vi "Check 2D Limits.vi"(2 "error in":T2, 4 "Z-Axis Communications Config":T1={"GPIB address"=22, "GPIB bus"=0, "connection ID"=refnum, "IP"="192.168.2.200", "Active Comm Interface"=0, "Serial Port"="", "Programmer Type"=0} {"Programmer Type" items=["Model 430", "Model 420"]; "Active Comm Interface" items=["TCP/IP (Model 430 Only)", "RS232", "IEEE488"]}, 5 "Y-Axis Communications Config":T1={"GPIB address"=22, "GPIB bus"=0, "connection ID"=refnum, "IP"="192.168.2.200", "Active Comm Interface"=0, "Serial Port"="", "Programmer Type"=0} {"Programmer Type" items=["Model 430", "Model 420"]; "Active Comm Interface" items=["TCP/IP (Model 430 Only)", "RS232", "IEEE488"]}, 6 "Z-Axis Field (T)":dbl format="%.3f", 7 "Y-Axis Field (T)":dbl format="%.3f") -> (0 "Within Limits?":bool, 1 "error out":T2)   [LabVIEW 2016]
uses:
  Instrument_Setup.vi
panel:
  out "Set Magnitude":dbl format="%#_13g"
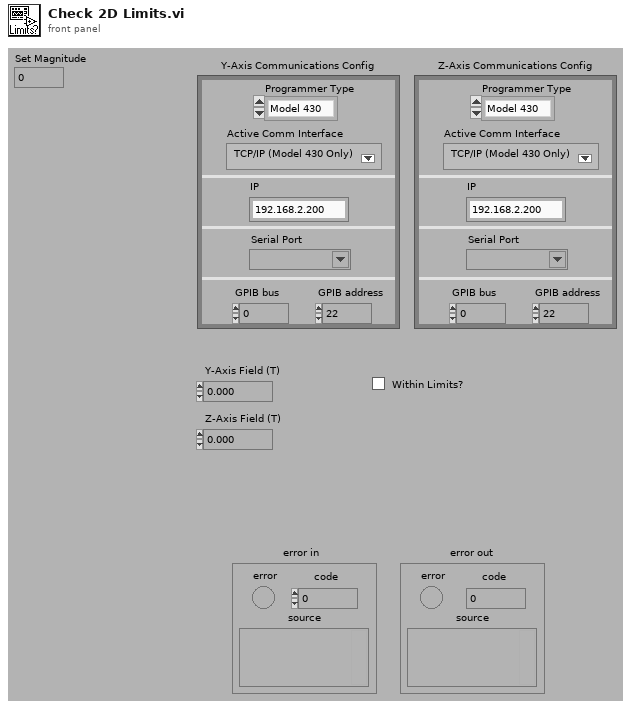
[diagram p1: front panel]
types:
  T1 = cluster{"GPIB address":i16, "GPIB bus":i16, "connection ID":refnum<k5>, "IP":string, "Active Comm Interface":u16, "Serial Port":refnum<visa-resource-name>, "Programmer Type":u16}
  T2 = cluster{"error":bool, "code":i32, "source":string}
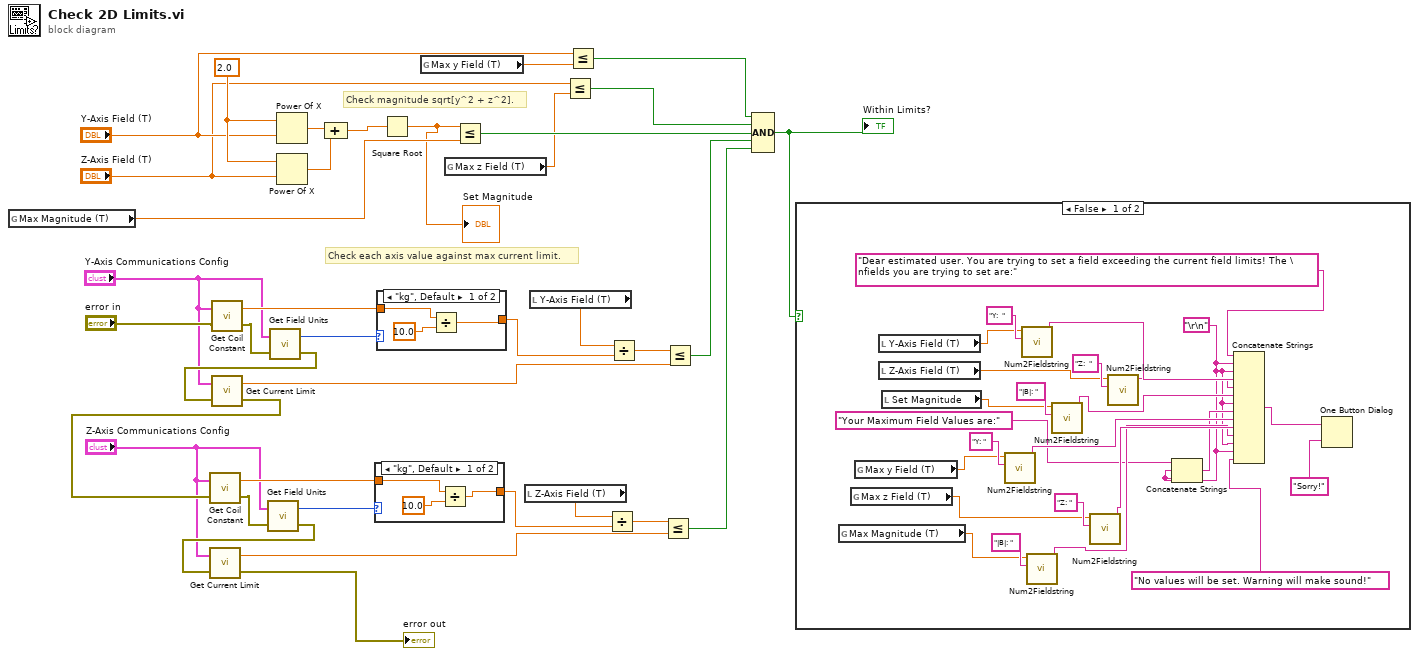
[diagram p0: block diagram]
diagram:
  w37 = 2.0 ("x")
  # "Check each axis value against max current limit."
  # "Check magnitude sqrt[y^2 + z^2]."
  n1 = global read "Instrument_Setup.vi" "Max Magnitude (T)"() -> (w5:dbl)
  n2 = call "Get Coil Constant.vi"("error in"="error in", "Communications Config"="Y-Axis Communications Config") -> ("error out"=w24:T2, "Coil Constant"=w25:dbl)
  n3 = call "Get Field Units.vi"("error in"=w24, "Z-Axis Communications Config"="Y-Axis Communications Config") -> ("error out"=w23:T2, "Field Units"=w26:enum16{"kg", "t"})
  n4 = call "Get Current Limit.vi"("error in"=w23, "Communications Config"="Y-Axis Communications Config") -> ("error out"=w18:T2, "Current Limit (A)"=w16:dbl)
  n5 = call "Get Coil Constant.vi"("error in"=w18, "Communications Config"="Z-Axis Communications Config") -> ("error out"=w20:T2, "Coil Constant"=w21:dbl)
  n6 = call "Get Field Units.vi"("error in"=w20, "Z-Axis Communications Config"="Z-Axis Communications Config") -> ("error out"=w19:T2, "Field Units"=w22:enum16{"kg", "t"})
  n7 = call "Get Current Limit.vi"("error in"=w19, "Communications Config"="Z-Axis Communications Config") -> ("error out"=→"error out":T2, "Current Limit (A)"=w14:dbl)
  n8 = Power Of X(1:"Y-Axis Field (T)", 2:w37) -> (0:w36:dbl)
  n9 = Power Of X(1:"Z-Axis Field (T)", 2:w37) -> (0:w35:dbl)
  n10 = Compound Arithmetic op=ADD(w36, w35) -> (w27:dbl)
  n11 = case shown="\"kg\", Default" w22 {
    tunnel: w21 -> [w39 w41]
    tunnel: [w38 w41] -> w15
    frame "kg", Default {
      n12 = Divide(x=w39, y=10.0) -> (x/y=w38:dbl)
    }
    frame "t" {
    }
  }
  n13 = case shown="\"kg\", Default" w26 {
    tunnel: w25 -> [w44 w45]
    tunnel: [w43 w45] -> w17
    frame "kg", Default {
      n14 = Divide(x=w44, y=10.0) -> (x/y=w43:dbl)
    }
    frame "t" {
    }
  }
  n15 = Square Root(x=w27) -> (sqrt(x)=w1:dbl)
  "Set Magnitude" <- w1
  n16 = global read "Instrument_Setup.vi" "Max y Field (T)"() -> (w3:dbl)
  n17 = global read "Instrument_Setup.vi" "Max z Field (T)"() -> (w4:dbl)
  n18 = Less Or Equal?(x=w1, y=w5) -> (x <= y?=w30:bool)
  n19 = local read "Z-Axis Field (T)"() -> (w31:dbl)
  n20 = local read "Y-Axis Field (T)"() -> (w34:dbl)
  n21 = Less Or Equal?(x="Z-Axis Field (T)", y=w4) -> (x <= y?=w6:bool)
  n22 = Less Or Equal?(x="Y-Axis Field (T)", y=w3) -> (x <= y?=w7:bool)
  n23 = Divide(x=w31, y=w15) -> (x/y=w32:dbl)
  n24 = Divide(x=w34, y=w17) -> (x/y=w33:dbl)
  n25 = Less Or Equal?(x=w32, y=w14) -> (x <= y?=w28:bool)
  n26 = Less Or Equal?(x=w33, y=w16) -> (x <= y?=w29:bool)
  n27 = Compound Arithmetic op=AND(w7, w6, w30, w29, w28) -> (w2:bool)
  "Within Limits?" <- w2
  n28 = case shown="False" w2 {
    frame False {
      w47 = "\r\n"
      n29 = global read "Instrument_Setup.vi" "Max Magnitude (T)"() -> (w62:dbl)
      n30 = global read "Instrument_Setup.vi" "Max z Field (T)"() -> (w63:dbl)
      n31 = global read "Instrument_Setup.vi" "Max y Field (T)"() -> (w64:dbl)
      n32 = local read "Y-Axis Field (T)"() -> (w59:dbl)
      n33 = local read "Z-Axis Field (T)"() -> (w60:dbl)
      n34 = local read "Set Magnitude"() -> (w61:dbl)
      n35 = call "Num2Fieldstring.vi"("String"="Y: ", "In"=w64) -> ("Out"=w54:string)  [unwired: 9 in]
      n36 = call "Num2Fieldstring.vi"("String"="Y:  ", "In"=w59) -> ("Out"=w57:string)  [unwired: 9 in]
      n37 = call "Num2Fieldstring.vi"("String"="|B|: ", "In"=w62) -> ("Out"=w52:string)  [unwired: 9 in]
      n38 = call "Num2Fieldstring.vi"("String"="|B|: ", "In"=w61) -> ("Out"=w55:string)  [unwired: 9 in]
      n39 = call "Num2Fieldstring.vi"("String"="Z: ", "In"=w63) -> ("Out"=w53:string)  [unwired: 9 in]
      n40 = call "Num2Fieldstring.vi"("String"="Z:  ", "In"=w60) -> ("Out"=w56:string)  [unwired: 9 in]
      n41 = Concatenate Strings("Your Maximum Field Values are:", w47, w47) -> (w48:string)
      n42 = Concatenate Strings("Dear estimated user. You are trying to set a field exceeding the current field limits! The \nfields you are trying to set are:", w47, w47, w57, w56, w55, w47, w48, w54, w53, w52, w47, w47, "No values will be set. Warning will make sound!") -> (w51:string)
      n43 = One Button Dialog(message=w51, button name ("OK")="Sorry!") -> ()  [unwired: 1 out]
    }
    frame True {
    }
  }
